vi "GenSolid.vi"(7 "Color":u32(colorbox), 11 "NumLeds":i32) -> (3 "Array":u32[](array[numeric]))   [LabVIEW 2018, in "ArduinoSerialBling.lvlib"]
uses:
  ArduinoSerialBling.lvlib
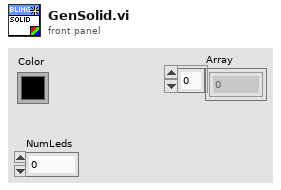
[diagram p1: front panel]
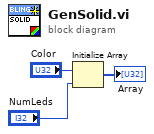
[diagram p0: block diagram]
diagram:
  n1 = Initialize Array("Color", "NumLeds") -> (→"Array":u32[])
